vi "Clean Up Actor.vi"(8 "error in (no error)":errorcluster, 11 "Terminal Message in":refnum<class "Terminal Message.lvclass">) -> (0 "error out":errorcluster, 3 "Terminal Message out":refnum<class "Terminal Message.lvclass">)   [LabVIEW 2016, in "CLD Exam - ATM.lvlib" / "Terminal Message.lvclass"]
uses:
  Terminal Message.lvclass
  D:/Repos/Stream/software/Mediator/Classes/Mediated Actor/Mediated Actor.lvclass
  Mediator/Classes/Message Broker Interface/Message Broker Interface.lvclass
  Mediator/Classes/Mediated Synchronous Actor/Mediated Synchronous Actor.lvclass
  Mediator/Classes/Mediated Actor/Mediated Actor.lvclass
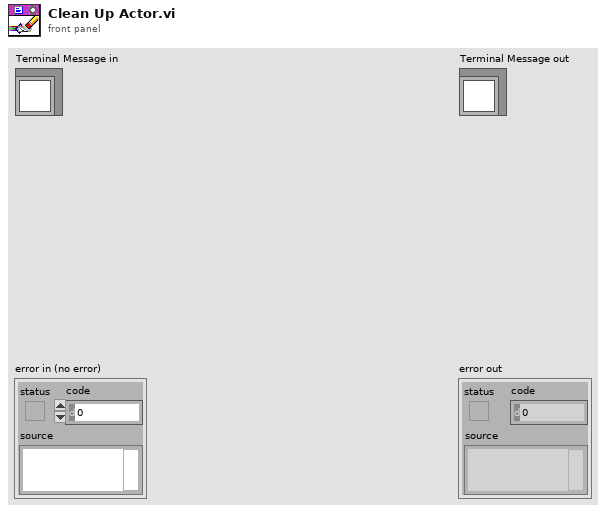
[diagram p1: front panel]
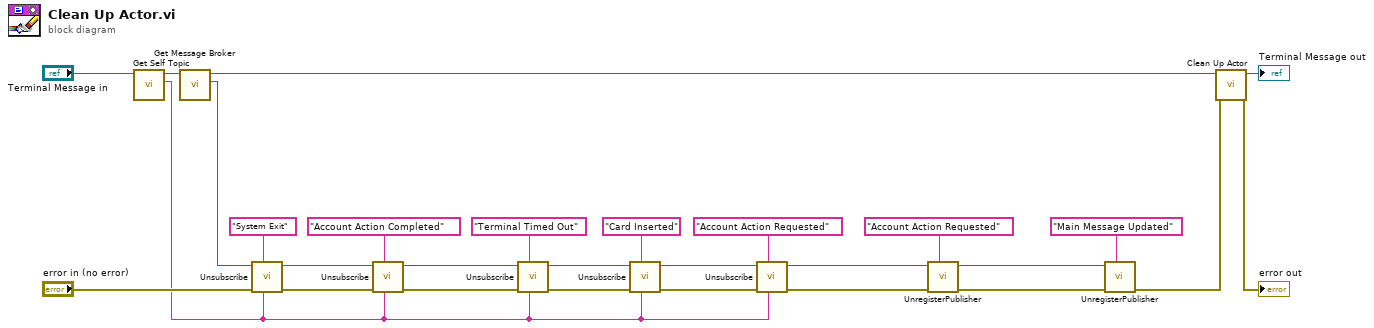
[diagram p0: block diagram]
diagram:
  n1 = call "Get Self Topic.vi"("Mediated Actor in"="Terminal Message in") -> ("Topic.Self"=w13:string, "Mediated Actor out"=w26:refnum<class "Terminal Message.lvclass">)  [unwired: 9 in]
  n2 = call "Get Message Broker.vi"("Mediated Actor in"=w26) -> ("Message Broker"=w20:refnum<class "Message Broker Interface.lvclass">, "Mediated Actor out"=w24:refnum<class "Terminal Message.lvclass">)  [unwired: 9 in]
  n3 = call-dynamic "Unsubscribe.vi"("Subscriber Name"=w13, "Topic Name"="System Exit", "error in (no error)"="error in (no error)", "Message Broker Interface in"=w20) -> ("error out"=w1:errorcluster, "Message Broker Interface out"=w2:refnum<class "Message Broker Interface.lvclass">)  [unwired: 6 in]
  n4 = call-dynamic "Unsubscribe.vi"("Subscriber Name"=w13, "Topic Name"="Account Action Completed", "error in (no error)"=w1, "Message Broker Interface in"=w2) -> ("error out"=w4:errorcluster, "Message Broker Interface out"=w3:refnum<class "Message Broker Interface.lvclass">)  [unwired: 6 in]
  n5 = call-dynamic "Unsubscribe.vi"("Subscriber Name"=w13, "Topic Name"="Terminal Timed Out", "error in (no error)"=w4, "Message Broker Interface in"=w3) -> ("error out"=w15:errorcluster, "Message Broker Interface out"=w16:refnum<class "Message Broker Interface.lvclass">)  [unwired: 6 in]
  n6 = call-dynamic "Unsubscribe.vi"("Subscriber Name"=w13, "Topic Name"="Card Inserted", "error in (no error)"=w15, "Message Broker Interface in"=w16) -> ("error out"=w11:errorcluster, "Message Broker Interface out"=w12:refnum<class "Message Broker Interface.lvclass">)  [unwired: 6 in]
  n7 = call-dynamic "Unsubscribe.vi"("Subscriber Name"=w13, "Topic Name"="Account Action Requested", "error in (no error)"=w11, "Message Broker Interface in"=w12) -> ("error out"=w7:errorcluster, "Message Broker Interface out"=w9:refnum<class "Message Broker Interface.lvclass">)  [unwired: 6 in]
  n8 = call-dynamic "UnregisterPublisher.vi"("Topic Name"="Account Action Requested", "error in (no error)"=w7, "Message Broker Interface in"=w9) -> ("error out"=w6:errorcluster, "Message Broker Interface out"=w8:refnum<class "Message Broker Interface.lvclass">)  [unwired: 7 in]
  n9 = call-dynamic "UnregisterPublisher.vi"("Topic Name"="Main Message Updated", "error in (no error)"=w6, "Message Broker Interface in"=w8) -> ("error out"=w5:errorcluster)  [unwired: 7 in, 1 out]
  n10 = call-parent "Clean Up Actor.vi"("error in (no error)"=w5, "Mediated Actor in"=w24) -> ("error out"=→"error out":errorcluster, "Mediated Actor out"=→"Terminal Message out":refnum<class "Terminal Message.lvclass">)  [unwired: 8 in]
